vi "Gyro Get Mode.vi"(8 "error in (no error)":errorcluster, 11 "I2CDevRef":T2={"DevStatus"={"status"=FALSE, "code"=0, "source"=""}, "Controller"=enum."Controller 1", "Device Address"=0, "Handle"=0, "I2C Bus"=enum."Invalid"} {"Device Address" format="%.0x"}) -> (0 "error out":errorcluster, 2 "DPS Mode":T1, 3 "I2CDevRef Out":T2={"DevStatus"={"status"=FALSE, "code"=0, "source"=""}, "Controller"=enum."Controller 1", "Device Address"=0, "Handle"=0, "I2C Bus"=enum."Invalid"} {"Device Address" format="%.0x"})   [LabVIEW 2014]
uses:
  <vilib>/Rock Robotics/WPI/I2C/WPI_I2CDevRef.ctl
  <vilib>/Rock Robotics/SystemInterfaces/Typedef/FPGA_TypedefDigitalModule.ctl
  <vilib>/Rock Robotics/SystemInterfaces/i2clib/i2c_bus.ctl
  DPS Mode.ctl
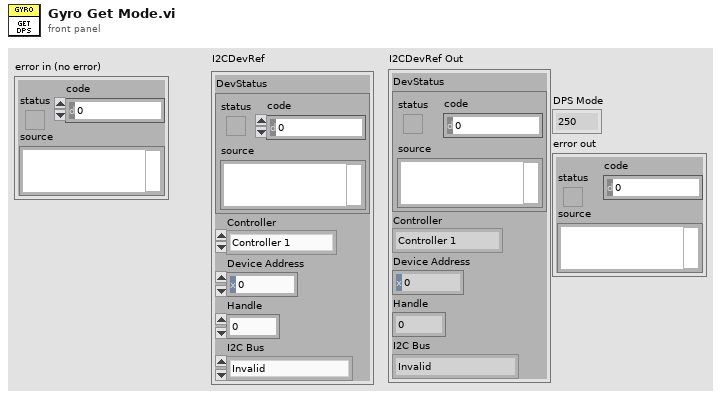
[diagram p1: front panel]
types:
  T1 = typedef "DPS Mode.ctl" = enum16{"250", "500", "2000"}
  T2 = typedef "WPI_I2CDevRef.ctl" = cluster{"DevStatus":errorcluster, "Controller":T3, "Device Address":u8, "Handle":i32, "I2C Bus":T4}
  T3 = typedef "FPGA_TypedefDigitalModule.ctl" = enum16{"Controller 1"}
  T4 = typedef "i2c_bus.ctl" = enum16{"I2C On-Board", "I2C MXP", "Invalid"}
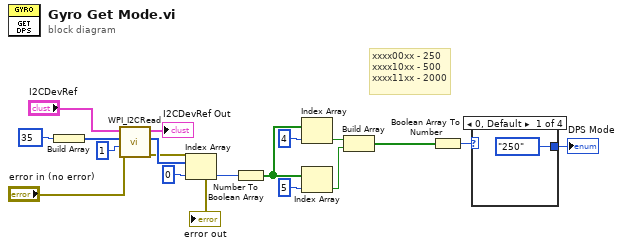
[diagram p0: block diagram]
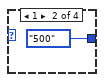
[diagram p2: hidden frame]
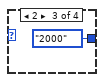
[diagram p3: hidden frame]
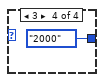
[diagram p4: hidden frame]
diagram:
  # "xxxx00xx - 250\nxxxx10xx - 500\nxxxx11xx - 2000"
  n1 = Build Array(u8 35 ("Data To Send")) -> (w12:u8[])
  n2 = call <vilib>:"WPI_I2CRead.vi"("error in (no error)"="error in (no error)", "I2CBytesToRead"=u8 1, "I2CRegister"=w12, "I2CDevRef"="I2CDevRef") -> ("error out"=→"error out":errorcluster, "Data Out"=w16:u8[], "I2CDevRef"=→"I2CDevRef Out":T2)  [unwired: 5 in]
  n3 = Index Array(array=w16, index=0) -> (element=w14:u8)
  n4 = Number To Boolean Array(number=w14) -> (Boolean array=w8:bool[])
  n5 = Index Array(array=w8, index=4) -> (element=w7:bool)
  n6 = Index Array(array=w8, index=5) -> (element=w6:bool)
  n7 = Build Array(w7, w6) -> (w5:bool[])
  n8 = Boolean Array To Number(Boolean array=w5) -> (number=w4:u32)
  n9 = case shown="0, Default" w4 {
    tunnel: [DPS_Mode."250" ("DPS Mode") DPS_Mode."500" ("DPS Mode") DPS_Mode."2000" ("DPS Mode") DPS_Mode."2000" ("DPS Mode")] -> w3
    frame 0, Default {
    }
    frame 1 {
    }
    frame 2 {
    }
    frame 3 {
    }
  }
  "DPS Mode" <- w3
